vi "Cal Value Global.vi"(8 "error in (no error)":errorcluster, 10 "Cal In":T1={"Calibrate?"=TRUE, "Scalling In "={"Raw Low "=1531.0, "Raw High"=6859.0, "Actual Low"=1.0, "Actual High"=4.9}}, 11 "Action":enum16{"Set", "Get "}(ring)) -> (0 "error out":errorcluster, 2 "Cal  Out":T1)   [LabVIEW 2023]
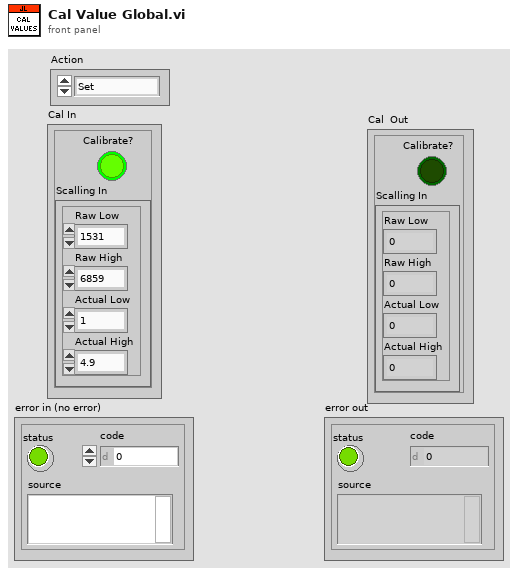
[diagram p1: front panel]
types:
  T1 = cluster{"Calibrate?":bool, "Scalling In ":cluster{"Raw Low ":dbl, "Raw High":dbl, "Actual Low":dbl, "Actual High":dbl}}
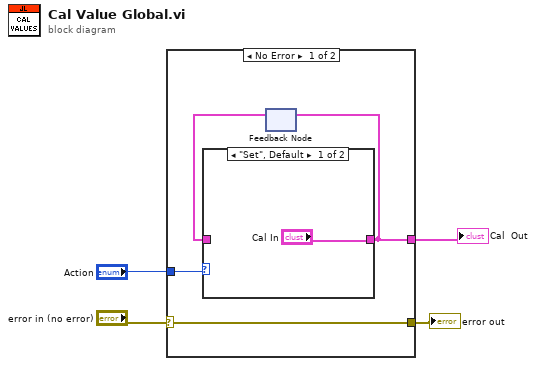
[diagram p0: block diagram]
diagram:
  n1 = case shown="No Error" "error in (no error)" {
    selector: "error in (no error)" -> [w7 w11]
    tunnel: [w7 w11] -> w3
    tunnel: "Action" -> [w6 _]
    tunnel: [w5 _] -> w1
    frame No Error {
      n2 = feedback #1() -> (w8:T1)  [unwired: 1 in]
      n3 = case shown="\"Set\", Default" w6 {
        tunnel: w8 -> [_ w10]
        tunnel: ["Cal In" w10] -> w5
        frame "Set", Default {
        }
        frame "Get " {
        }
      }
      n4 = feedback-in #1(w5) -> ()
    }
    frame Error {
    }
  }
  "error out" <- w3
  "Cal  Out" <- w1
